vi "Sub_2016_05_04_SinBias.vi"(8 "Number of steps":dbl=5.0, 9 "Start current":dbl=55.0, 11 "Finish current":dbl=100.0) -> (0 "Array 2":dbl[](array[numeric]), 3 "Array":dbl[](array[numeric])=[55.0, 61.59009742330268, 77.5, 93.40990257669732, 100.0])   [LabVIEW 2015]
panel:
  out "Waveform Graph":dbl[](graph)
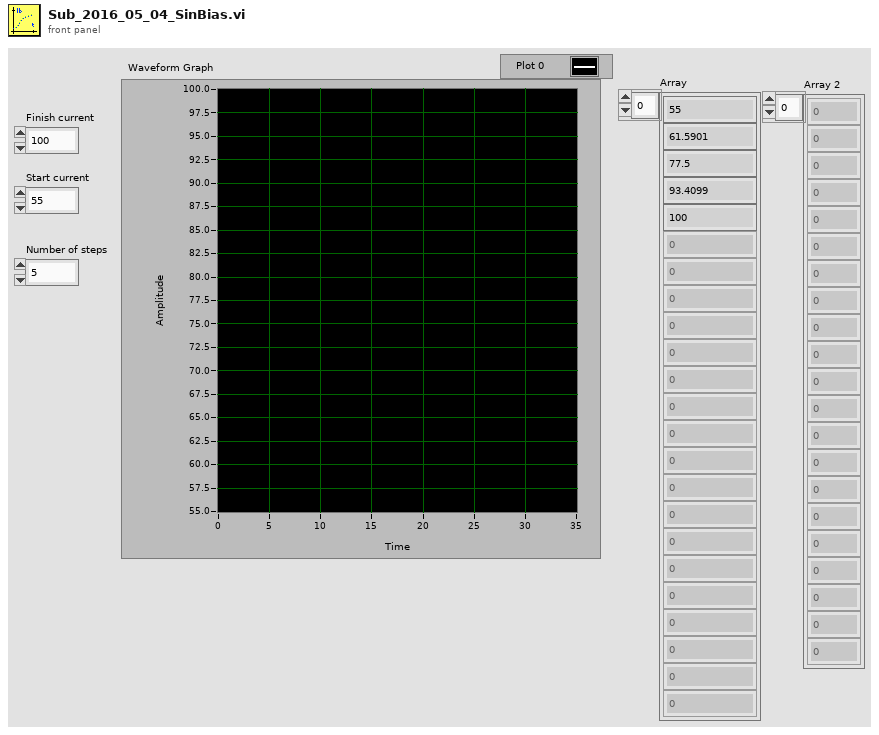
[diagram p1: front panel]
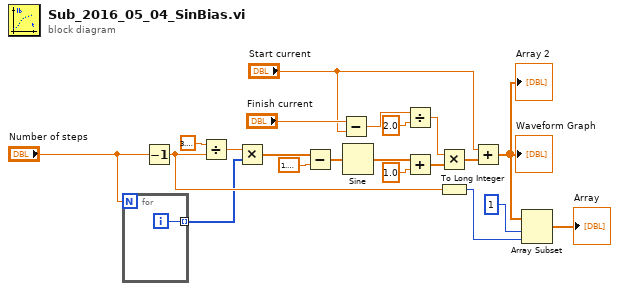
[diagram p0: block diagram]
diagram:
  n1 = for {
    N: "Number of steps" -> [_]
    tunnel: [w22] -> w2 mode=indexing
    i -> [w22]
  }
  n2 = Decrement(x="Number of steps") -> (x-1=w18:dbl)
  n3 = Divide(x=3.141592653589793, y=w18) -> (x/y=w5:dbl)
  n4 = Multiply(x=w5, y=w2) -> (x*y=w11:dbl[])
  n5 = Subtract(x=w11, y=1.5707963267948966) -> (x-y=w9:dbl[])
  n6 = Subtract(x="Finish current", y="Start current") -> (x-y=w3:dbl)
  n7 = Sine(x=w9) -> (sin(x)=w14:dbl[])
  n8 = Divide(x=w3, y=2.0) -> (x/y=w6:dbl)
  n9 = Add(x=w14, y=1.0) -> (x+y=w12:dbl[])
  n10 = Multiply(x=w6, y=w12) -> (x*y=w8:dbl[])
  n11 = To Long Integer(number=w18) -> (32bit integer=w17:i32)
  n12 = Add(x="Start current", y=w8) -> (x+y=w1:dbl[])
  "Waveform Graph" <- w1
  "Array 2" <- w1
  n13 = Array Subset(array=w1, index=1, length=w17) -> (→"Array":dbl[])
